vi "Point.vi"(8 "错误输入":errorcluster caption="错误输入（无错误）", 10 "Point":T1[](array[typedef]), 11 "Step":enum16{"Initial", "Write", "Read"}(ring)) -> (0 "错误输出":errorcluster, 2 "Point":T1[](array[typedef]))   [LabVIEW 2017]
uses:
  Ctrls/Point.ctl
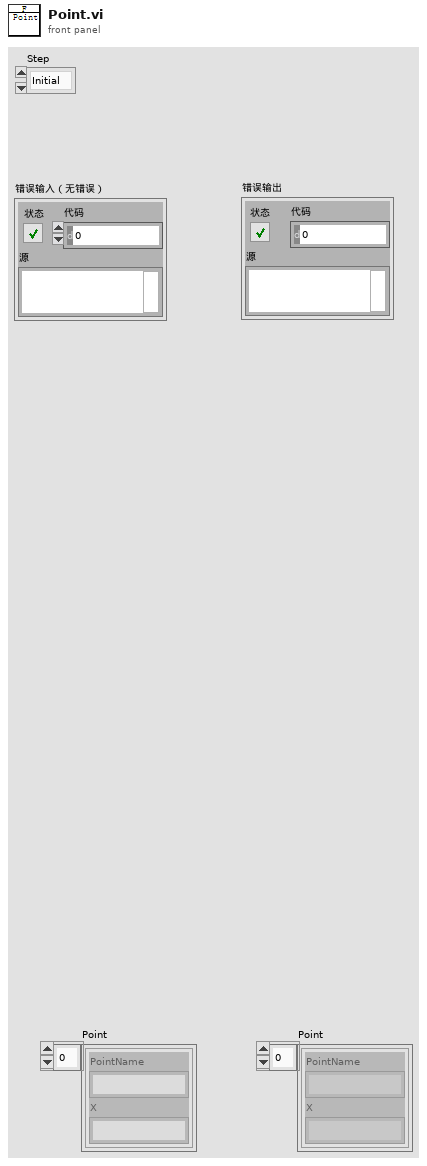
[diagram p1: front panel]
types:
  T1 = typedef "Point.ctl" = cluster{"PointName":string, "X":string}
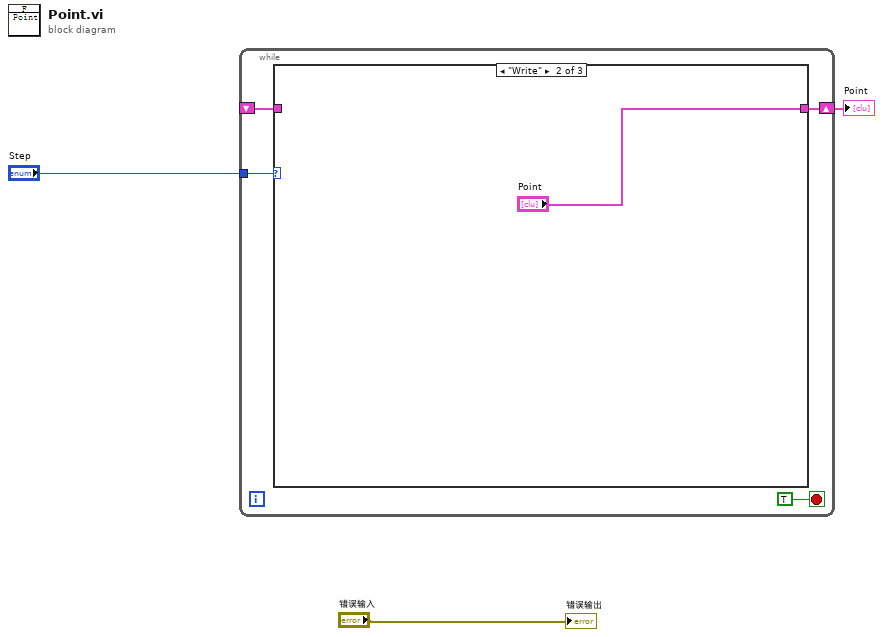
[diagram p0: block diagram]
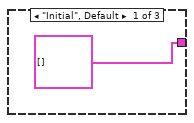
[diagram p2: hidden frame]
diagram:
  n1 = while {
    tunnel: "Step" -> [w6]
    shift-right: [w5] -> w1
    shift-left: _ -> [w4]
    stop <- TRUE stop-if-true
    n2 = case shown="\"Write\"" w6 {
      tunnel: [cluster{"PointName":string, "X":string}[] [] "Point" w10] -> w5
      tunnel: w4 -> [_ _ w10]
      frame "Initial", Default {
      }
      frame "Write" {
      }
      frame "Read" {
      }
    }
  }
  "Point" <- w1
  "错误输出" <- "错误输入"
